vi "Cmd_U32U32U32U32U32U8.vi"(0 "VISA Refnum in":refnum<visa-resource-name>, 1 "Arg1":u32 max=127 step=1, 2 "Arg2":u32 max=127 step=1, 3 "Arg3":u32, 5 "Address":u8, 7 "Cmd":u8, 8 "Arg4":u32, 10 "Arg5":u32, 11 "error in (no error)":errorcluster, 14 "Arg6":u8) -> (4 "VISA Refnum out":refnum<visa-resource-name>, 6 "Valid":bool, 15 "error out":errorcluster)   [LabVIEW 2015, in "Ion Motion Roboclaw.lvlib"]
uses:
  <instrlib>/Ion Motion Roboclaw/Ion Motion Roboclaw.lvlib
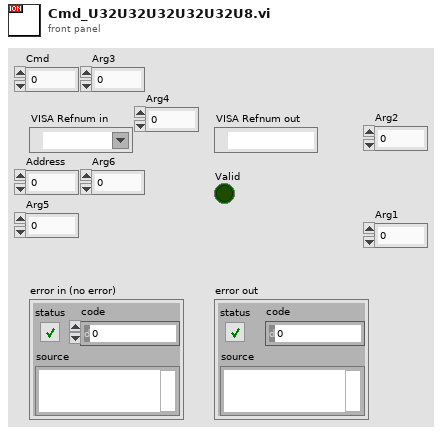
[diagram p1: front panel]
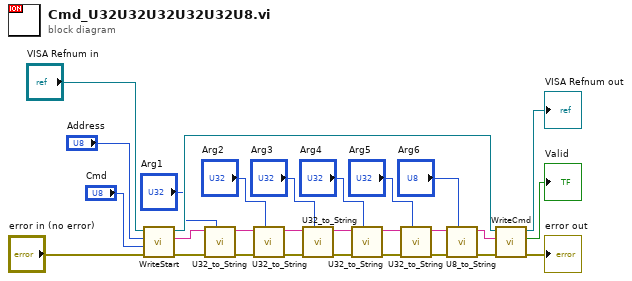
[diagram p0: block diagram]
diagram:
  n1 = call <instrlib>:"WriteStart.vi"("error in (no error)"="error in (no error)", "Cmd"="Cmd", "Address"="Address", "VISA Refnum in"="VISA Refnum in") -> ("error out"=w20:errorcluster, "String Out"=w21:string, "VISA Refnum out"=w23:refnum<visa-resource-name>)  [unwired: 5 in]
  n2 = call <instrlib>:"U32_to_String.vi"("number"="Arg1", "error in (no error)"=w20, "String In"=w21) -> ("error out"=w19:errorcluster, "String Out"=w18:string)  [unwired: 5 in]
  n3 = call <instrlib>:"U32_to_String.vi"("number"="Arg2", "error in (no error)"=w19, "String In"=w18) -> ("error out"=w13:errorcluster, "String Out"=w14:string)  [unwired: 5 in]
  n4 = call <instrlib>:"U32_to_String.vi"("number"="Arg3", "error in (no error)"=w13, "String In"=w14) -> ("error out"=w11:errorcluster, "String Out"=w10:string)  [unwired: 5 in]
  n5 = call <instrlib>:"U32_to_String.vi"("number"="Arg4", "error in (no error)"=w11, "String In"=w10) -> ("error out"=w3:errorcluster, "String Out"=w5:string)  [unwired: 5 in]
  n6 = call <instrlib>:"U32_to_String.vi"("number"="Arg5", "error in (no error)"=w3, "String In"=w5) -> ("error out"=w2:errorcluster, "String Out"=w4:string)  [unwired: 5 in]
  n7 = call <instrlib>:"U8_to_String.vi"("Argument"="Arg6", "error in (no error)"=w2, "String In"=w4) -> ("error out"=w7:errorcluster, "String Out"=w8:string)  [unwired: 5 in]
  n8 = call <instrlib>:"WriteCmd.vi"("error in (no error)"=w7, "write buffer"=w8, "VISA Refnum in"=w23) -> ("error out"=→"error out":errorcluster, "Valid"=→"Valid":bool, "VISA Refnum out"=→"VISA Refnum out":refnum<visa-resource-name>)  [unwired: 2 in]
